vi "post_dust_event_big.vi"(8 "error in (no error)":errorcluster, 10 "Signal Array":T1[](array[typedef]), 11 "Cluster":T4 {"File Location" items=["Unknown"=-1, "Storage"=0, "Processing"=1]}) -> (0 "error out":errorcluster, 1 "Experiment Settings":i32, 2 "Dust Event ID":i64)   [LabVIEW 2015]
uses:
  User Interface/Controls/Post_Dust_Event.ctl
  User Interface/Controls/File_location.ctl
  User Interface/Controls/Signal.ctl
  User Interface/Controls/Role ID.ctl
  User Interface/Controls/Hardware ID.ctl
  NaN_screening_big.vi
  <vilib>/addons/database/_DB Variant To Data/Database Variant To Data.xnode
panel:
  # "Signal"
  # "Dust Event"
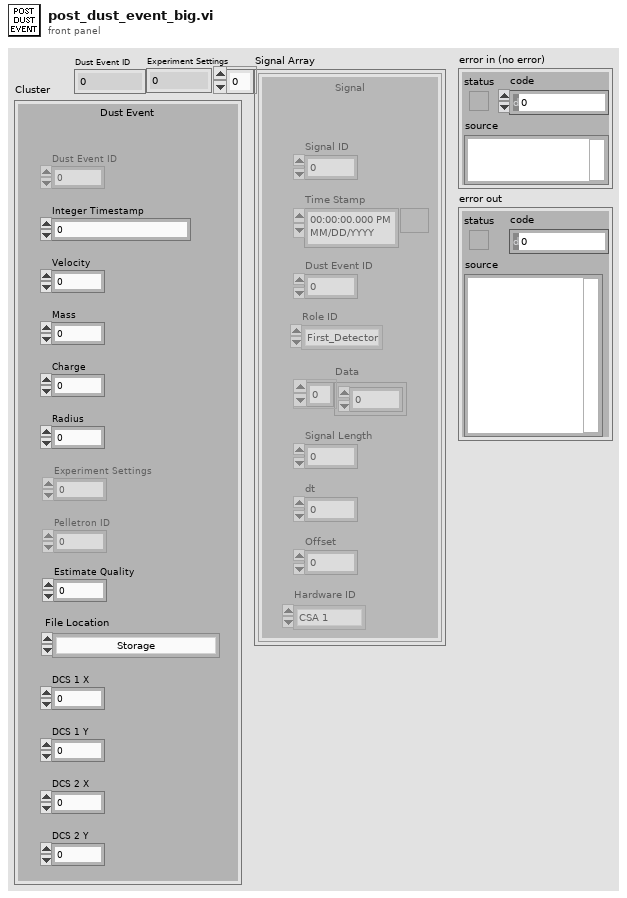
[diagram p1: front panel]
types:
  T1 = typedef "Signal.ctl" = cluster{"Signal ID":i64, "Time Stamp":timestamp, "Dust Event ID":i64, "Role ID":T2, "Data":sgl[], "Signal Length":i32, "dt":sgl, "Offset":dbl, "Hardware ID":T3}
  T2 = typedef "Role ID.ctl" = enum16{"First_Detector", "Second_Detector", "Third_Detector", "LeCroy_CH1", "LeCroy_CH2", "LeCroy_CH3", "LeCroy_CH4", "PSU", "DCS 1", "DCS 2"}
  T3 = typedef "Hardware ID.ctl" = enum16{"Unknown", "CSA 1", "CSA 2", "CSA 3", "CSA 4", "CSA 5", "CSA 6", "DCS 1", "DCS 2"}
  T4 = typedef "Post_Dust_Event.ctl" = cluster{"Dust Event ID":i64, "Integer Timestamp":i64, "Velocity":sgl, "Mass":sgl, "Charge":sgl, "Radius":sgl, "Experiment Settings":dbl, "Pelletron ID":i32, "Estimate Quality":sgl, "File Location":T5, "id_dust_info":dbl, "DCS 1 X":sgl, "DCS 1 Y":sgl, "DCS 2 X":sgl, "DCS 2 Y":sgl}
  T5 = typedef "File_location.ctl" = i8
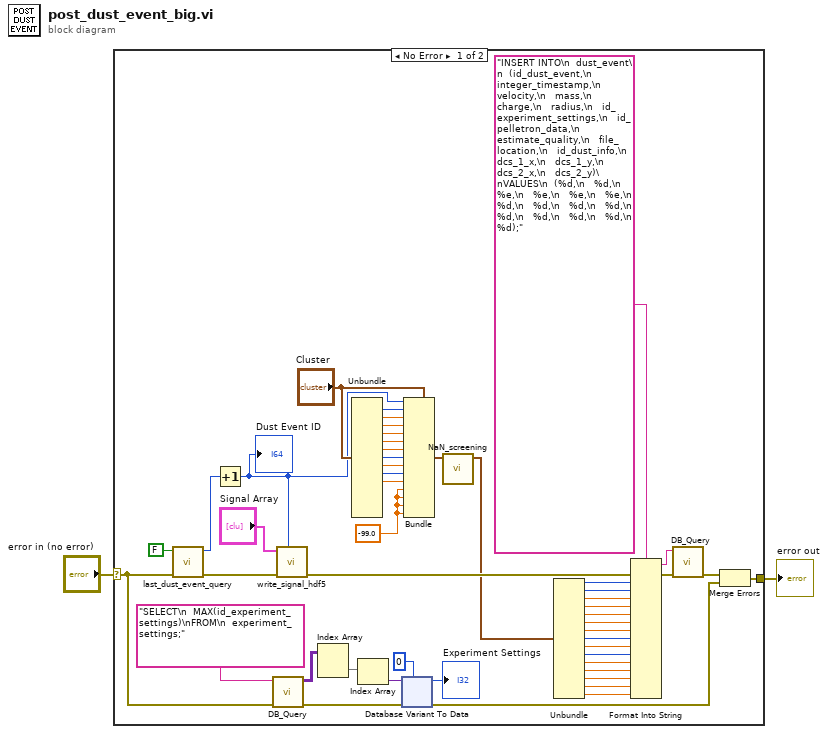
[diagram p0: block diagram]
diagram:
  n1 = case shown="No Error" "error in (no error)" {
    selector: "error in (no error)" -> [w29 w84]
    tunnel: [w51 w84] -> w1
    frame No Error {
      w27 = sgl -99.0 ("DCS 2 Y")
      n2 = call "last_dust_event_query.vi"("error in (no error)"=w29, "Small?"=FALSE) -> ("error out"=w35:errorcluster, "id_dust_event"=w34:i64)  [unwired: 8 in]
      n3 = Increment(x=w34) -> (x+1=w38:i64)
      "Dust Event ID" <- w38
      n4 = call "DB_Query.vi"("error in (no error)"=w29, "Parameterized Query"="SELECT\n  MAX(id_experiment_settings)\nFROM\n  experiment_settings;" ("SQL query")) -> ("error out"=w32:errorcluster, "Results"=w30:variant[][])  [unwired: 7 in, 1 out]
      n5 = call "write_signal_hdf5.vi"("Index"=w38, "error in"=w35, "Signal array"="Signal Array") -> ("error out"=w21:errorcluster)  [unwired: 7 in, 1 out]
      n6 = Index Array(array=w30) -> (element=w25:variant[])  [unwired: 2 in]
      n7 = Unbundle("Cluster") -> ("Integer Timestamp"=w39:i64, "Velocity"=w40:sgl, "Mass"=w41:sgl, "Charge"=w42:sgl, "Radius"=w43:sgl, "Experiment Settings"=w44:dbl, "Pelletron ID"=w45:i32, "Estimate Quality"=w46:sgl, "File Location"=w37:T5, "id_dust_info"=w47:dbl)  [unwired: 5 out]
      n8 = Index Array(array=w25) -> (element=w24:variant)  [unwired: 1 in]
      n9 = xnode "Database Variant To Data"("database variant"=w24, "error in (no error)"=w32, "type"=0) -> ("data"=→"Experiment Settings":i32, "error out"=w31:errorcluster)
      n10 = Bundle(cluster="Cluster", "Dust Event ID"=w38, "Integer Timestamp"=w39, "Velocity"=w40, "Mass"=w41, "Charge"=w42, "Radius"=w43, "Experiment Settings"=w44, "Pelletron ID"=w45, "Estimate Quality"=w46, "File Location"=w37, "id_dust_info"=w47, "DCS 1 X"=w27, "DCS 1 Y"=w27, "DCS 2 X"=w27, "DCS 2 Y"=w27) -> (w48:T4)
      n11 = call-poly "NaN_screening.vi"("Input"=w48) -> ("Output"=w18:T4)  [unwired: 10 in]
      n12 = Unbundle(w18) -> ("Dust Event ID"=w17:i64, "Integer Timestamp"=w3:i64, "Velocity"=w4:sgl, "Mass"=w5:sgl, "Charge"=w6:sgl, "Radius"=w7:sgl, "Experiment Settings"=w8:dbl, "Pelletron ID"=w9:i32, "Estimate Quality"=w10:sgl, "File Location"=w11:T5, "id_dust_info"=w12:dbl, "DCS 1 X"=w13:sgl, "DCS 1 Y"=w14:sgl, "DCS 2 X"=w15:sgl, "DCS 2 Y"=w16:sgl)
      n13 = Format Into String(format string="INSERT INTO\n  dust_event\n  (id_dust_event,\n   integer_timestamp,\n   velocity,\n   mass,\n   charge,\n   radius,\n   id_experiment_settings,\n   id_pelletron_data,\n   estimate_quality,\n   file_location,\n   id_dust_info,\n   dcs_1_x,\n   dcs_1_y,\n   dcs_2_x,\n   dcs_2_y)\nVALUES\n  (%d,\n   %d,\n   %e,\n   %e,\n   %e,\n   %e,\n   %d,\n   %d,\n   %d,\n   %d,\n   %d,\n   %d,\n   %d,\n   %d,\n   %d);" ("Parameterized Query"), error in=w21, w17, w3, w4, w5, w6, w7, w8, w9, w10, w11, w12, w13, w14, w15, w16) -> (resulting string=w19:string, error out=w20:errorcluster)  [unwired: 1 in]
      n14 = call "DB_Query.vi"("error in (no error)"=w20, "Parameterized Query"=w19) -> ("error out"=w23:errorcluster)  [unwired: 7 in, 2 out]
      n15 = Merge Errors(w23, w31) -> (w51:errorcluster)
    }
    frame Error {
    }
  }
  "error out" <- w1
